vi "Example Plots.vi"() -> ()   [LabVIEW 2019, in "LcWebView.lvclass"]
uses:
  LcWebView.lvclass
  C:/Projects/WebView2/LcWebView/data/Microsoft.Web.WebView2.WinForms.dll
panel:
  out "Status Message":string
  out "Status":i32(ring) items=["Created", "WaitingForActivation", "WaitingToRun", "Running", "WaitingForChildrenToComplete", "RanToCompletion", "Canceled", "Faulted"]
  out "Initialise Loops":i32
  in  "Web 4":refnum<k24>(container)
  in  "Web 3":refnum<k24>(container)
  in  "Web 2":refnum<k24>(container)
  in  "stop":bool
  in  "Web":refnum<k24>(container)
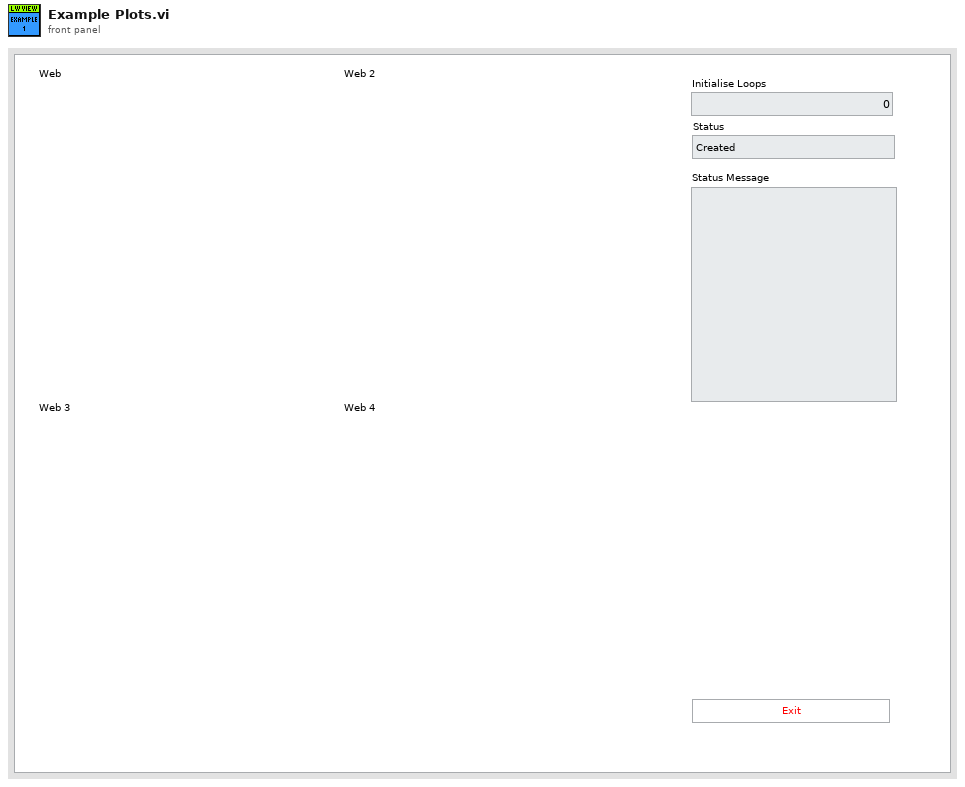
[diagram p1: front panel]
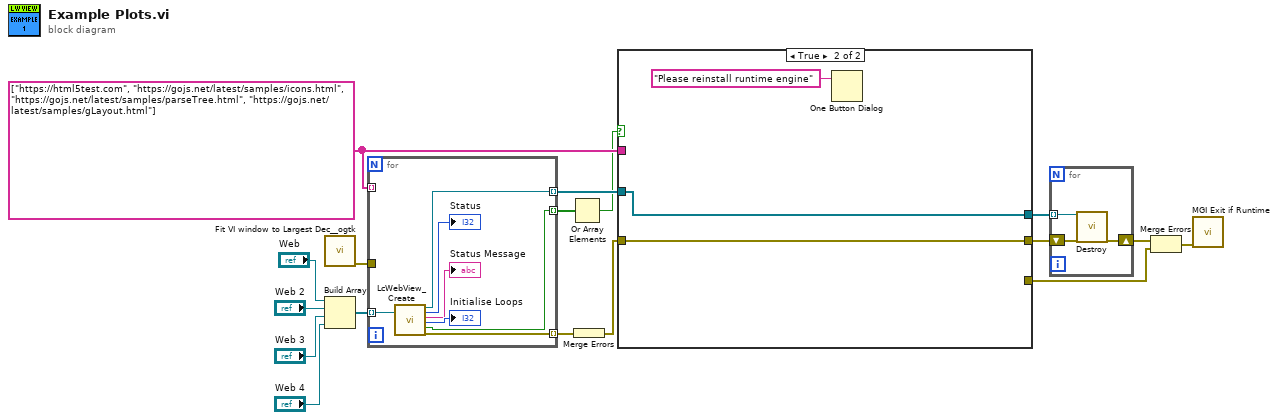
[diagram p0: block diagram]
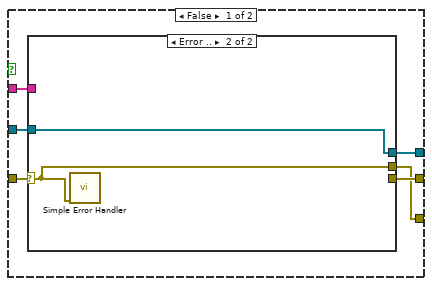
[diagram p2: hidden frame]
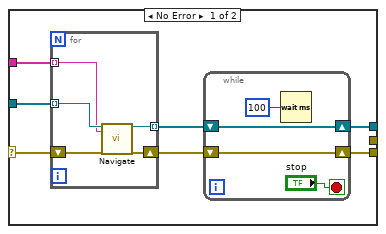
[diagram p3: hidden frame]
diagram:
  w10 = string[] ["https://html5test.com", "https://gojs.net/latest/samples/icons.html", "https://gojs.net/latest/samples/parseTree.html", "https://gojs.net/latest/samples/gLayout.html"] ("URL")
  n1 = call "Fit VI window to Largest Dec__ogtk.vi"() -> ("error out"=w2:errorcluster)  [unwired: 6 in, 1 out]
  n2 = Build Array("Web", "Web 2", "Web 3", "Web 4") -> (w6:refnum<k24>[])
  n3 = for {
    tunnel: [w24] -> w17 mode=indexing
    tunnel: [w23] -> w16 mode=indexing
    tunnel: [w22] -> w11 mode=indexing
    tunnel: w10 -> [_] mode=indexing
    tunnel: w6 -> [w21] mode=indexing
    tunnel: w2 -> [_]
    n4 = call "LcWebView_Create.vi"("Webview container"=w21) -> ("reference out"=w24:refnum<class "LcWebView.lvclass">, "Status"=→"Status":i32, "Status Message"=→"Status Message":string, "Initialise Loops"=→"Initialise Loops":i32, "Reinstall Runtime"=w22:bool, "Error Out"=w23:errorcluster)  [unwired: 11 in, 2 out]
  }
  n5 = Or Array Elements(Boolean array=w11) -> (logical OR=w3:bool)
  n6 = Merge Errors(w16) -> (w5:errorcluster)
  n7 = case shown="True" w3 {
    tunnel: w17 -> [w30 w51]
    tunnel: w5 -> [w29 w50]
    tunnel: [w28 w51] -> w15
    tunnel: [w27 w50] -> w14
    tunnel: [w26 _] -> w12
    tunnel: w10 -> [w25 _]
    frame False {
      n8 = case shown="Error .." w29 {
        selector: w29 -> [w36 w47]
        tunnel: w30 -> [w37 w48]
        tunnel: [w33 w48] -> w28
        tunnel: [w32 _] -> w27
        tunnel: [_ w47] -> w26
        tunnel: w25 -> [w31 _]
        frame No Error {
          n9 = for {
            tunnel: w37 -> [w42] mode=indexing
            tunnel: [w40] -> w35 mode=indexing
            shift-right: [w39] -> w34
            shift-left: w36 -> [w41]
            tunnel: w31 -> [w38] mode=indexing
            n10 = call-dynamic "Navigate.vi"("reference in"=w42, "URL"=w38, "Error In"=w41) -> ("reference out"=w40:refnum<class "LcWebView.lvclass">, "Error Out"=w39:errorcluster)  [unwired: 14 in, 1 out]
          }
          n11 = while {
            shift-right: [w45] -> w33
            shift-left: w35 -> [w45]
            shift-right: [w44] -> w32
            shift-left: w34 -> [w44]
            stop <- "stop" stop-if-true
            n12 = Wait (ms)(milliseconds to wait=u32 100) -> ()  [unwired: 1 out]
          }
        }
        frame Error {
          n13 = call <vilib>:"Simple Error Handler.vi"("error in (no error)"=w47) -> ()  [unwired: 4 in, 5 out]
        }
      }
    }
    frame True {
      n14 = One Button Dialog(message="Please reinstall runtime engine") -> ()  [unwired: 1 in, 1 out]
    }
  }
  n15 = for {
    tunnel: w15 -> [w54] mode=indexing
    shift-right: [w52] -> w13
    shift-left: w14 -> [w53]
    n16 = call-dynamic "Destroy.vi"("reference in"=w54, "Error In"=w53) -> ("Error Out"=w52:errorcluster)  [unwired: 16 in, 1 out]
  }
  n17 = Merge Errors(w13, w12) -> (w1:errorcluster)
  n18 = call "MGI Exit if Runtime.vi"("Error In (Dependency Only)"=w1) -> ()  [unwired: 11 in]
